vi "MM Command to Cntrl Loop Actuator In.vi"(0 "Target":T2[](array[typedef]), 5 "Current Cartesian Position":dbl[][](array[numeric]), 7 "Number of\nLBCBs In":T1, 11 "error in (no error)":errorcluster, 13 "Rigid Connection":bool) -> (6 "Cmd Out":T3[](array[typedef]), 15 "error out":errorcluster)   [LabVIEW 2013]
uses:
  Act & Cart Commands.ctl
  MixedMode/Target Data.ctl
  Data Access Objects/Application/Number Of LBCBs.ctl
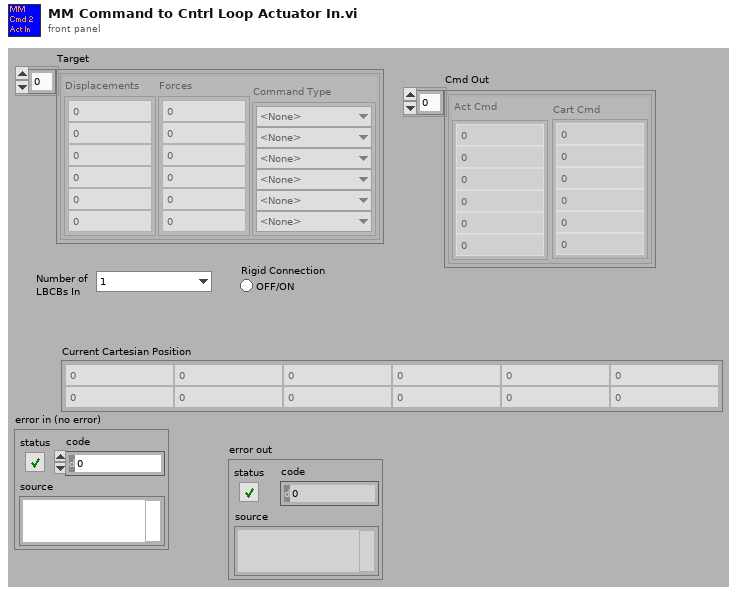
[diagram p1: front panel]
types:
  T1 = typedef "Number Of LBCBs.ctl" = enum16{"1", "2"}
  T2 = typedef "Target Data.ctl" = cluster{"Displacements":dbl[], "Command Type":enum16{"<None>", "Displacement", "Force"}[], "Forces":dbl[]}
  T3 = typedef "Act & Cart Commands.ctl" = cluster{"Act Cmd":dbl[], "Cart Cmd":dbl[]}
  T4 = enum16{"Cartesian2ActuatorDisplacements", "Actuator2CartesianDisplacements", "Actuators2CartesianForces"}
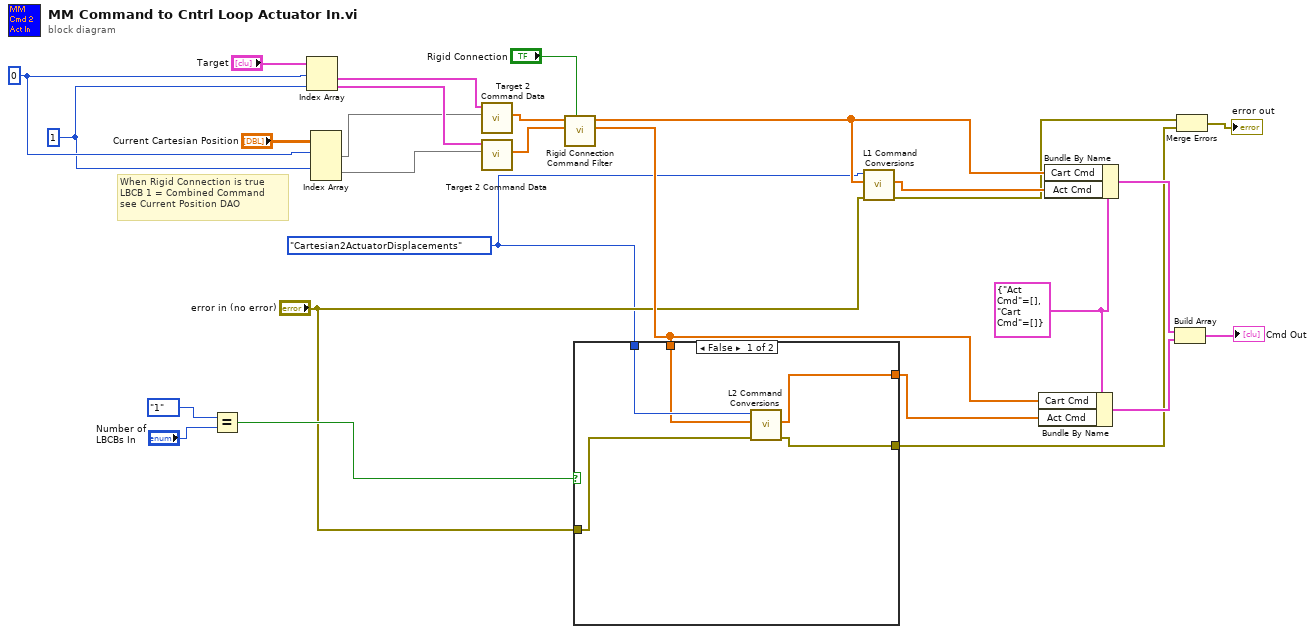
[diagram p0: block diagram]
diagram:
  w3 = T4."Cartesian2ActuatorDisplacements" ("ConversionOps")
  w19 = T3 {"Act Cmd"=[], "Cart Cmd"=[]} ("element")
  w13 = 1 ("index (row)")
  w14 = 0 ("index (row)")
  # "When Rigid Connection is true\nLBCB 1 = Combined Command\nsee Current Position DAO"
  n1 = Equal?(x=Number_Of_LBCBs."1", y="Number of\nLBCBs In") -> (x = y?=w8:bool)
  n2 = Index Array(array="Target", index #1=w14, index #2=w13) -> (element #1=w24:T2, element #2=w23:T2)
  n3 = Index Array(array="Current Cartesian Position", index (row) #1=w14, index (row) #2=w13) -> (element #1=w12:dbl[], element #2=w11:dbl[])  [unwired: 2 in]
  n4 = call "Target 2 Command Data.vi"("Current \nPosition"=w12, "Command Data"=w24) -> ("Output"=w18:dbl[])  [unwired: 9 out]
  n5 = call "Target 2 Command Data.vi"("Current \nPosition"=w11, "Command Data"=w23) -> ("Output"=w17:dbl[])  [unwired: 9 out]
  n6 = call "Rigid Connection Command Filter.vi"("Rigid Connection"="Rigid Connection", "LBCB 2 Commands In"=w17, "LBCB 1 Commands In"=w18) -> ("LBCB 2 Commands Out"=w7:dbl[], "LBCB 1 Commands Out"=w4:dbl[])  [unwired: 7 in]
  n7 = case shown="False" w8 {
    tunnel: w7 -> [w31 w34]
    tunnel: [w28 w34] -> w9
    tunnel: "error in (no error)" -> [w30 w33]
    tunnel: [w29 w33] -> w6
    tunnel: w3 -> [w32 _]
    frame False {
      n8 = call "L2 Command Conversions.vi"("error in (no error)"=w30, "Inputs"=w31, "ConversionOps"=w32) -> ("error out"=w29:errorcluster, "Outputs"=w28:dbl[])  [unwired: 7 in]
    }
    frame True {
    }
  }
  n9 = call "L1 Command Conversions.vi"("error in (no error)"="error in (no error)", "Inputs"=w4, "ConversionOps"=w3) -> ("error out"=w1:errorcluster, "Outputs"=w2:dbl[])  [unwired: 7 in]
  n10 = Bundle By Name(cluster=w19, "Cart Cmd"=w7, "Act Cmd"=w9) -> (w21:T3)
  n11 = Bundle By Name(cluster=w19, "Cart Cmd"=w4, "Act Cmd"=w2) -> (w22:T3)
  n12 = Build Array(w22, w21) -> (→"Cmd Out":T3[])
  n13 = Merge Errors(w1, w6) -> (→"error out":errorcluster)
